vi "Draw Shapes.vi"(6 "Output Point":T1, 8 "Results":T2, 9 "new picture in":picture, 10 "Points":cluster{"x":dbl, "y":dbl, "th":dbl}[](array[cluster]), 11 "Picture in":refnum<vi>) -> (3 "new picture out":picture)   [LabVIEW 2019]
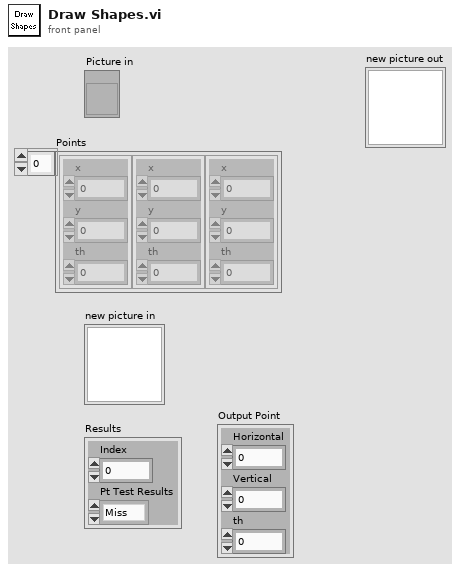
[diagram p1: front panel]
types:
  T1 = cluster{"Horizontal":dbl, "Vertical":dbl, "th":dbl}
  T2 = cluster{"Index":i32, "Pt Test Results":enum16{"Miss", "Rect Hit", "Arrow Hit"}}
  T3 = cluster{i32, "Pt Test Results":enum16{"Miss", "Rect Hit", "Arrow Hit"}}
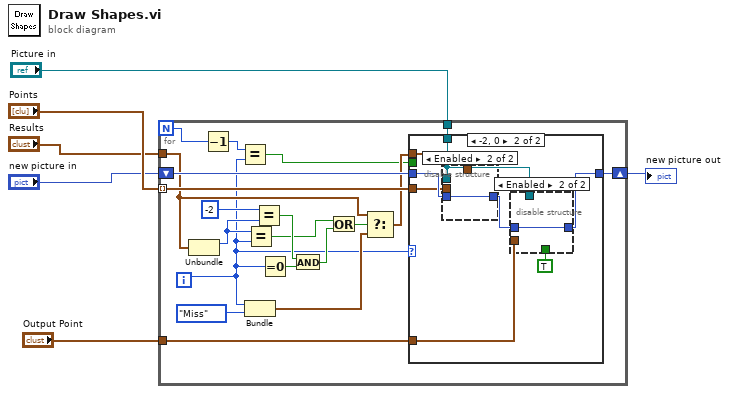
[diagram p0: block diagram]
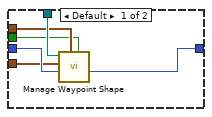
[diagram p2: hidden frame]
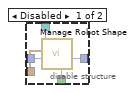
[diagram p3: hidden frame]
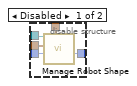
[diagram p4: hidden frame]
diagram:
  n1 = for {
    N -> [w11]
    tunnel: "Points" -> [w26] mode=indexing
    shift-right: [w25] -> w4
    shift-left: "new picture in" -> [w24]
    tunnel: "Picture in" -> [w23]
    tunnel: "Results" -> [w20]
    tunnel: "Output Point" -> [w7]
    i -> [w9]
    n2 = Unbundle(w20) -> ("Index"=w16:i32)  [unwired: 1 out]
    n3 = Decrement(x=w11) -> (x-1=w10:i32)
    n4 = Equal?(x=w10, y=w9) -> (x = y?=w8:bool)
    n5 = Bundle(w9, "Pt Test Results"=enum16{"Miss", "Rect Hit", "Arrow Hit"}."Miss") -> (w21:T3)  [unwired: 1 in]
    n6 = Equal?(x=w16, y=w9) -> (x = y?=w13:bool)
    n7 = Equal?(x=-2, y=w16) -> (x = y?=w15:bool)
    n8 = Equal To 0?(x=w9) -> (x = 0?=w18:bool)
    n9 = And(x=w15, y=w18) -> (x .and. y?=w14:bool)
    n10 = Or(x=w13, y=w14) -> (x .or. y?=w12:bool)
    n11 = Select(t=w20, s=w12, f=w21) -> (s? t:f=w22:T2)
    n12 = case shown="-2, 0" w9 {
      tunnel: w26 -> [w28 w39]
      tunnel: [w31 w37] -> w25
      tunnel: w24 -> [w32 w40]
      tunnel: w23 -> [w30 w35]
      tunnel: w22 -> [w29 w38]
      tunnel: w8 -> [w27 _]
      tunnel: w7 -> [_ w36]
      frame Default {
        n13 = call "Manage Waypoint Shape.vi"("Draw Arrow"=w27, "Drawing Options"=w29, "new picture in"=w32, "Waypoint Position (ft)"=w28, "Pict Ref"=w30) -> ("new picture out"=w31:picture)  [unwired: 5 in, 1 out]
      }
      frame -2, 0 {
        n14 = disable-structure shown="Enabled" {
          disable-tunnel: w40 -> [w51 w52]
          disable-tunnel: w39 -> [w50 _]
          disable-tunnel: w38 -> [w49 _]
          disable-tunnel: w35 -> [w48 _]
          disable-tunnel: [w47 w52] -> w34
          frame Disabled {
            n15 = call "Manage Robot Shape.vi"("Drawing Options"=w49, "new picture in"=w51, "Robot Position (ft)"=w50, "Pict Ref"=w48) -> ("new picture out"=w47:picture)  [unwired: 5 in, 2 out]
          }
          frame Enabled {
          }
        }
        n16 = disable-structure shown="Enabled" {
          disable-tunnel: [w45 w46] -> w37
          disable-tunnel: w36 -> [w44 _]
          disable-tunnel: w35 -> [w43 _]
          disable-tunnel: w34 -> [w42 w46]
          disable-tunnel: TRUE ("Outline") -> [w41 _]
          frame Disabled {
            n17 = call "Manage Robot Shape.vi"("Lighter"=w41, "new picture in"=w42, "Robot Position (ft)"=w44, "Pict Ref"=w43) -> ("new picture out"=w45:picture)  [unwired: 5 in, 2 out]
          }
          frame Enabled {
          }
        }
      }
    }
  }
  "new picture out" <- w4
